vi "Start Chassis.vi"(5 "Cfg wChassis":T1, 6 "Show FP?":bool, 7 "Actor-to-Caller Enqueuer":refnum<class "Message Enqueuer.lvclass">, 8 "error in (no error)":errorcluster, 9 "TCP LS Writer":refnum<class "Message Enqueuer.lvclass">, 10 "TCP HS Writer":refnum<class "Message Enqueuer.lvclass">, 11 "HS Only in":refnum<class "HS Only.lvclass">) -> (0 "error out":errorcluster, 3 "HS Only out":refnum<class "HS Only.lvclass">)   [LabVIEW 2012, in "Data Acquisition.lvlib" / "HS Only.lvclass"]
uses:
  HS Only.lvclass
  <vilib>/ActorFramework/Message Enqueuer/Message Enqueuer.lvclass
  Custom Ctrls/Master Cfg/ge_Cfg wChassis.ctl
  Cfg Grandmaster/Class Chassis BOM/Chassis BOM.lvclass
  Cfg Grandmaster/Class Chassis Cfg/ChassisCfg.lvclass
  Class Chassis Tasks/Chassis Tasks.lvclass
  Common/Controls/TE_Designator.ctl
  Class DAQ Actor/DAQ Actor.lvclass
  Class Chassis Tasks/Chassis Tasks.lvclass/Chassis Tasks.ctl
  <vilib>/ActorFramework/Message Enqueuer/Message Enqueuer.lvclass/Message Enqueuer.ctl
  Class Chassis Tasks/Read HS DAQ Task.vi
  Class Chassis Tasks/Write HS ActorQ.vi
  <vilib>/ActorFramework/Message Enqueuer/Enqueue.vi
  <vilib>/ActorFramework/Message Priority Queue/Priority Enqueue.vi
  Class DAQ Task/DAQ Task.lvclass
  DAQ Actor Messages/Start Task Msg/Start Task Msg.lvclass
  <vilib>/ActorFramework/Actor/Actor.lvclass
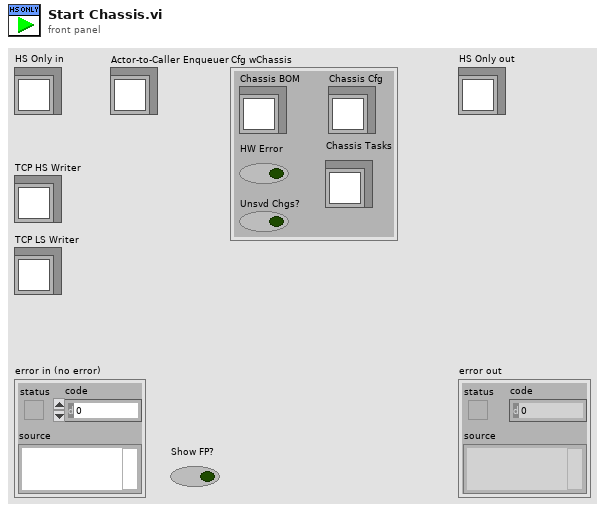
[diagram p1: front panel]
types:
  T1 = typedef "ge_Cfg wChassis.ctl" = cluster{"Chassis BOM":refnum<class "Chassis BOM.lvclass">, "Chassis Cfg":refnum<class "ChassisCfg.lvclass">, "Chassis Tasks":refnum<class "Chassis Tasks.lvclass">, "HW Error":bool, "Unsvd Chgs?":bool}
  T2 = typedef "TE_Designator.ctl" = enum16{"High Speed", "Low Speed"}
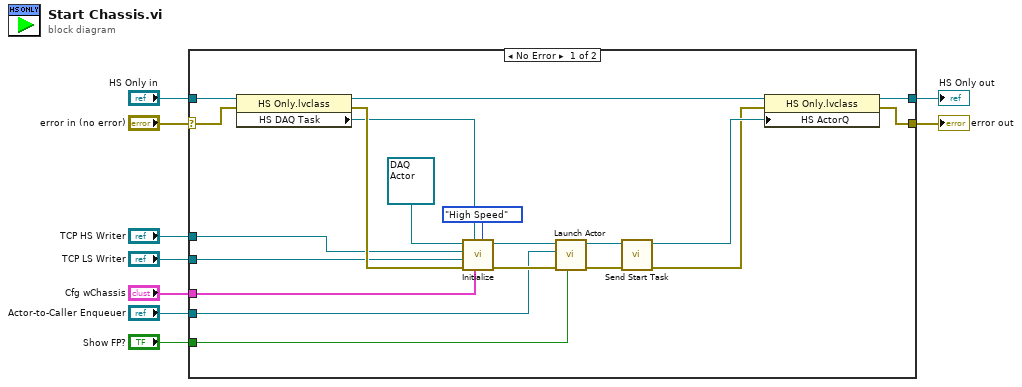
[diagram p0: block diagram]
diagram:
  n1 = case shown="No Error" "error in (no error)" {
    selector: "error in (no error)" -> [w16 w31]
    tunnel: "Actor-to-Caller Enqueuer" -> [w26 _]
    tunnel: "Cfg wChassis" -> [w12 _]
    tunnel: [w23 w30] -> w7
    tunnel: [w22 w31] -> w6
    tunnel: "HS Only in" -> [w21 w30]
    tunnel: "TCP HS Writer" -> [w18 _]
    tunnel: "TCP LS Writer" -> [w17 _]
    tunnel: "Show FP?" -> [w10 _]
    frame No Error {
      n2 = property class="HS Only.lvclass"(reference=w21, error in=w16) -> (reference out=w20:refnum<class "HS Only.lvclass">, error out=w19:errorcluster, "HS DAQ Task"=w13:refnum<class "DAQ Task.lvclass">)
      n3 = call-dynamic "Initialize.vi"("TimingEngine"=TE_Designator."High Speed", "Cfg wChassis"=w12, "LS DAQ Task"=w13, "error in (no error)"=w19, "TCP LS Writer"=w17, "TCP HS Writer"=w18, "DAQ Actor in"=refnum<class "DAQ Actor.lvclass"> refnum) -> ("error out"=w29:errorcluster, "DAQ Actor out"=w28:refnum<class "DAQ Actor.lvclass">)  [unwired: 3 in]
      n4 = call <vilib>:"Launch Actor.vi"("Open Actor Core front panel? (F)"=w10, "error in (no error)"=w29, "Actor-to-Caller Enqueuer"=w26, "Actor"=w28) -> ("error out"=w24:errorcluster, "Caller-To-Actor Enqueuer"=w25:refnum<class "Message Enqueuer.lvclass">)  [unwired: 6 in]
      n5 = call "Send Start Task.vi"("error in (no error)"=w24, "Message Enqueuer"=w25) -> ("error out"=w14:errorcluster, "Message Enqueuer out"=w15:refnum<class "Message Enqueuer.lvclass">)  [unwired: 8 in]
      n6 = property class="HS Only.lvclass"(reference=w20, error in=w14, "HS ActorQ"=w15) -> (reference out=w23:refnum<class "HS Only.lvclass">, error out=w22:errorcluster)
    }
    frame Error {
    }
  }
  "error out" <- w6
  "HS Only out" <- w7
